vi "N-Channel N-Samples (2D DBL).vi"() -> ()   [LabVIEW 2020]
uses:
  <vilib>/DAQmx/read.llb/DAQmx Read (Analog 2D DBL NChan NSamp).vi
  <vilib>/DAQmx/create/channels.llb/DAQmx Create Channel (AI-Voltage-Basic).vi
  <vilib>/DAQmx/configure/timing.llb/DAQmx Timing (Sample Clock).vi
  <vilib>/DAQmx/miscellaneous.llb/DAQmx Fill In Error Info.vi
  <resource>/objmgr/daqmx.rc
panel:
  out "Actual Sample Rate (Hz)":dbl
  in  "Desired Sample Rate (Hz)":dbl=2560.0
  in  "Number of Samples":i32=256
  in  "Stop":bool
  in  "Physical Channels":tag
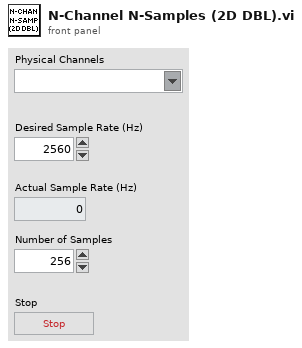
[diagram p1: front panel]
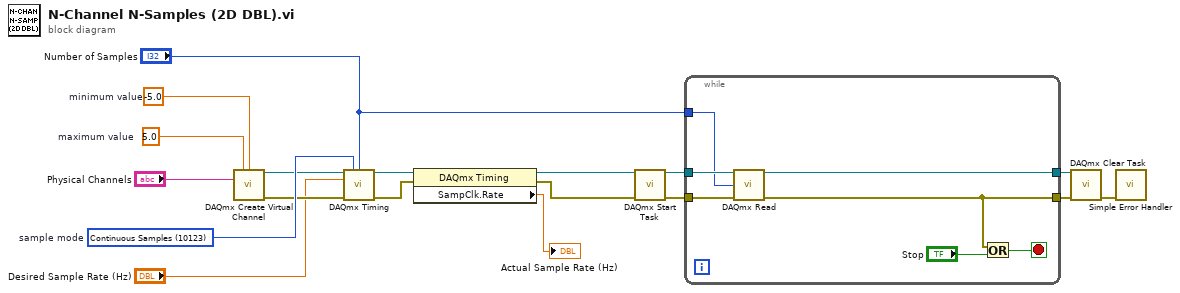
[diagram p0: block diagram]
diagram:
  w13 = 5.0  # maximum value
  w14 = -5.0  # minimum value
  w18 = 10123 items=["Finite Samples"=10178, "Continuous Samples"=10123, "Hardware Timed Single Point"=12522]  # sample mode
  n1 = call-poly <vilib>:"DAQmx Create Virtual Channel.vi"("maximum value"=w13, "minimum value"=w14, "physical channels"="Physical Channels") -> ("task out"=w17:refnum<k21>, "error out"=w16:errorcluster)  [unwired: 11 in]
  n2 = call-poly <vilib>:"DAQmx Timing.vi"("task/channels in"=w17, "sample mode"=w18, "samples per channel"="Number of Samples", "rate"="Desired Sample Rate (Hz)", "error in"=w16) -> ("task out"=w5:refnum<k21>, "error out"=w4:errorcluster)  [unwired: 9 in]
  n3 = property class="DAQmx Timing"(reference=w5, error in=w4) -> (reference out=w3:refnum<k21>, error out=w2:errorcluster, "SampClk.Rate"=→"Actual Sample Rate (Hz)":dbl)
  n4 = call <vilib>:"DAQmx Start Task.vi"("task/channels in"=w3, "error in"=w2) -> ("task out"=w9:refnum<k21>, "error out"=w8:errorcluster)  [unwired: 12 in]
  n5 = while {
    tunnel: [w25] -> w12
    tunnel: [w24] -> w11
    tunnel: w9 -> [w21]
    tunnel: w8 -> [w20]
    tunnel: "Number of Samples" -> [w19]
    stop <- w22 stop-if-true
    n6 = call-poly <vilib>:"DAQmx Read.vi"("task/channels in"=w21, "number of samples per channel"=w19, "error in"=w20) -> ("task out"=w25:refnum<k21>, "error out"=w24:errorcluster)  [unwired: 10 in, 1 out]
    n7 = Or(x=w24, y="Stop") -> (x .or. y?=w22:bool)
  }
  n8 = call <vilib>:"DAQmx Clear Task.vi"("task in"=w12, "error in"=w11) -> ("error out"=w10:errorcluster)  [unwired: 13 in]
  n9 = call <vilib>:"Simple Error Handler.vi"("error in (no error)"=w10) -> ()  [unwired: 4 in, 5 out]
